vi "PIDBoundaries.vi"(0 "SetPointIn":dbl[](array[numeric]), 1 "EncPosIn":dbl[](array[numeric]), 2 "BndrsCluster":T2, 3 "PIDGainsIn":T1, 4 "EncMax":dbl[](array[numeric])) -> (5 "SetPointOut":dbl[](array[numeric]), 6 "PIDGainsOut":T3(array[cluster]))   [LabVIEW 2013]
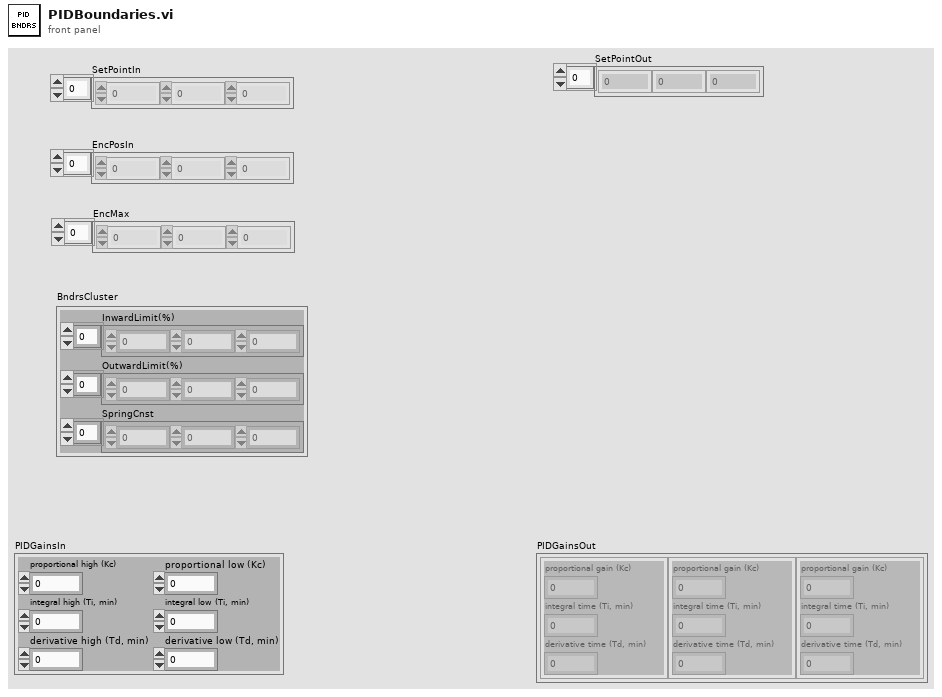
[diagram p1: front panel]
types:
  T1 = cluster{"proportional high (Kc)":dbl, "integral high (Ti, min)":dbl, "derivative high (Td, min)":dbl, "derivative low (Td, min)":dbl, "integral low (Ti, min)":dbl, "proportional low (Kc)":dbl}
  T2 = cluster{"InwardLimit(%)":dbl[], "OutwardLimit(%)":dbl[], "SpringCnst":dbl[]}
  T3 = cluster{"proportional gain (Kc)":dbl, "integral time (Ti, min)":dbl, "derivative time (Td, min)":dbl}[]
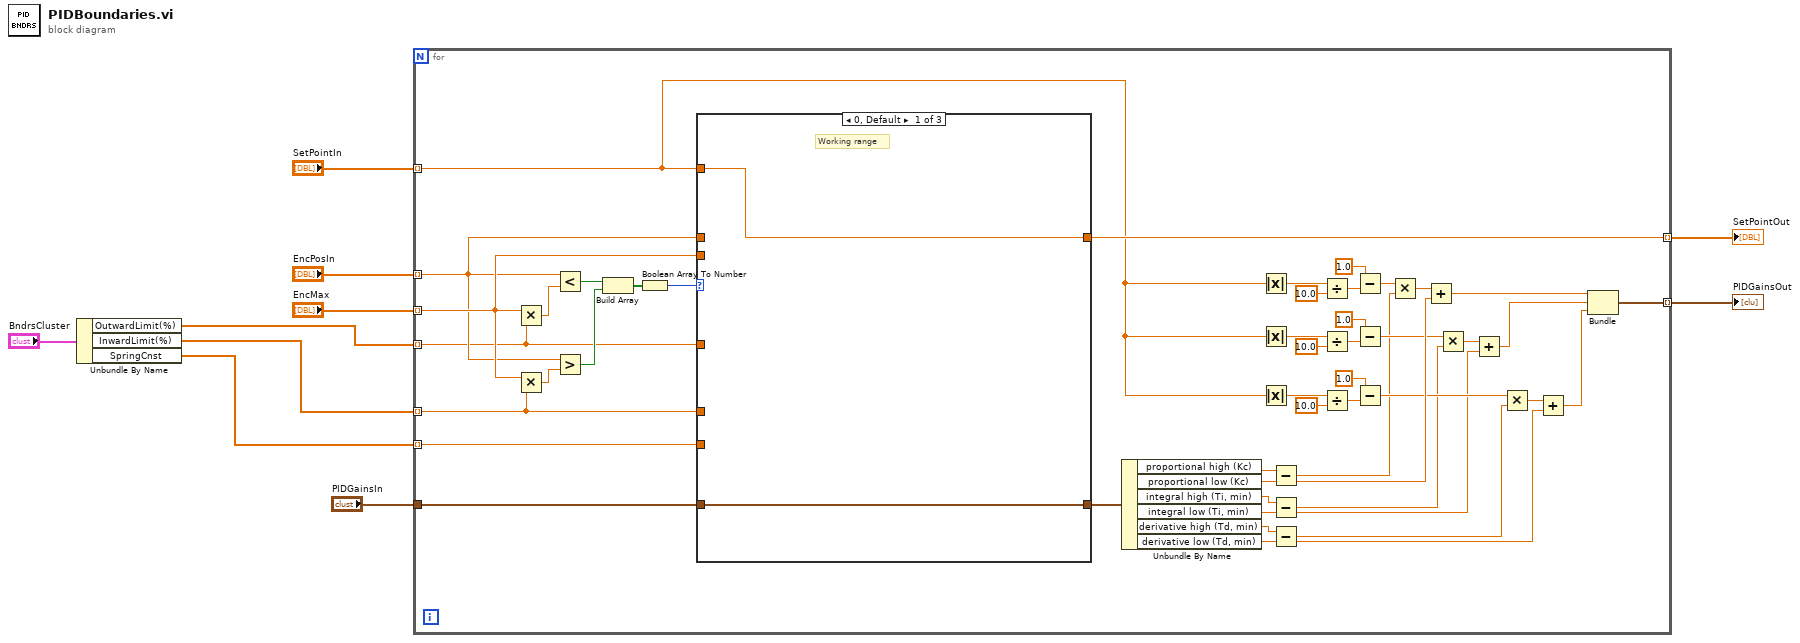
[diagram p0: block diagram]
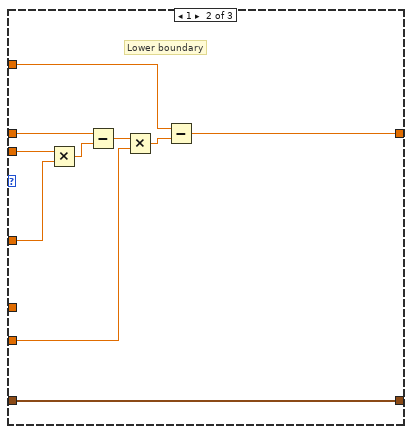
[diagram p2: hidden frame]
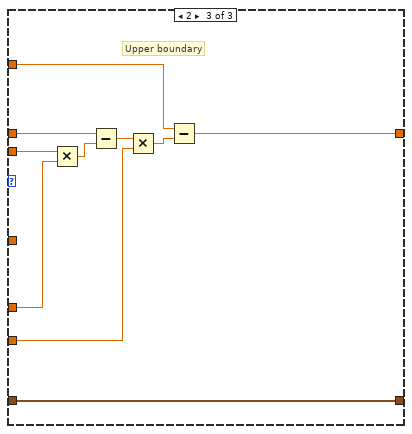
[diagram p3: hidden frame]
diagram:
  n1 = Unbundle By Name("BndrsCluster") -> ("OutwardLimit(%)"=w6:dbl[], "InwardLimit(%)"=w5:dbl[], "SpringCnst"=w4:dbl[])
  n2 = for {
    tunnel: "SetPointIn" -> [w22] mode=indexing
    tunnel: "EncMax" -> [w51] mode=indexing
    tunnel: "EncPosIn" -> [w50] mode=indexing
    tunnel: [w44] -> w10 mode=indexing
    tunnel: w6 -> [w49] mode=indexing
    tunnel: w5 -> [w48] mode=indexing
    tunnel: w4 -> [w47] mode=indexing
    tunnel: "PIDGainsIn" -> [w46]
    tunnel: [w11] -> w1 mode=indexing
    n3 = Multiply(x=w51, y=w49) -> (x*y=w56:dbl)
    n4 = Multiply(x=w51, y=w48) -> (x*y=w55:dbl)
    n5 = Less?(x=w50, y=w56) -> (x < y?=w54:bool)
    n6 = Greater?(x=w50, y=w55) -> (0:w53:bool)
    n7 = Build Array(w54, w53) -> (w52:bool[])
    n8 = Boolean Array To Number(Boolean array=w52) -> (number=w45:u32)
    n9 = case shown="0, Default" w45 {
      tunnel: [w57 w60 w70] -> w44
      tunnel: w22 -> [w57 w65 w77]
      tunnel: w50 -> [_ w64 w74]
      tunnel: w51 -> [_ w63 w73]
      tunnel: w46 -> [w58 w59 w69]
      tunnel: [w58 w59 w69] -> w38
      tunnel: w47 -> [_ w62 w72]
      tunnel: w49 -> [_ w61 _]
      tunnel: w48 -> [_ _ w71]
      frame 0, Default {
        # "Working range"
      }
      frame 1 {
        # "Lower boundary"
        n10 = Multiply(x=w63, y=w61) -> (x*y=w68:dbl)
        n11 = Subtract(x=w64, y=w68) -> (x-y=w67:dbl)
        n12 = Multiply(x=w67, y=w62) -> (x*y=w66:dbl)
        n13 = Subtract(x=w65, y=w66) -> (x-y=w60:dbl)
      }
      frame 2 {
        # "Upper boundary"
        n14 = Multiply(x=w73, y=w71) -> (x*y=w78:dbl)
        n15 = Subtract(x=w74, y=w78) -> (x-y=w76:dbl)
        n16 = Multiply(x=w76, y=w72) -> (x*y=w75:dbl)
        n17 = Subtract(x=w77, y=w75) -> (x-y=w70:dbl)
      }
    }
    n18 = Unbundle By Name(w38) -> ("proportional high (Kc)"=w37:dbl, "proportional low (Kc)"=w35:dbl, "integral high (Ti, min)"=w20:dbl, "integral low (Ti, min)"=w17:dbl, "derivative high (Td, min)"=w19:dbl, "derivative low (Td, min)"=w15:dbl)
    n19 = Absolute Value(x=w22) -> (abs(x)=w43:dbl)
    n20 = Absolute Value(x=w22) -> (abs(x)=w28:dbl)
    n21 = Absolute Value(x=w22) -> (abs(x)=w27:dbl)
    n22 = Subtract(x=w37, y=w35) -> (x-y=w21:dbl)
    n23 = Subtract(x=w20, y=w17) -> (x-y=w18:dbl)
    n24 = Subtract(x=w19, y=w15) -> (x-y=w16:dbl)
    n25 = Divide(x=w43, y=10.0) -> (x/y=w41:dbl)
    n26 = Divide(x=w28, y=10.0) -> (x/y=w30:dbl)
    n27 = Divide(x=w27, y=10.0) -> (x/y=w25:dbl)
    n28 = Subtract(x=1.0, y=w41) -> (x-y=w39:dbl)
    n29 = Subtract(x=1.0, y=w30) -> (x-y=w32:dbl)
    n30 = Subtract(x=1.0, y=w25) -> (x-y=w23:dbl)
    n31 = Multiply(x=w39, y=w21) -> (x*y=w36:dbl)
    n32 = Add(x=w36, y=w35) -> (x+y=w34:dbl)
    n33 = Multiply(x=w32, y=w18) -> (x*y=w33:dbl)
    n34 = Add(x=w33, y=w17) -> (x+y=w14:dbl)
    n35 = Multiply(x=w23, y=w16) -> (x*y=w13:dbl)
    n36 = Add(x=w13, y=w15) -> (x+y=w12:dbl)
    n37 = Bundle(w34, w14, w12) -> (w11:cluster{dbl, dbl, dbl})  [unwired: 1 in]
  }
  "SetPointOut" <- w10
  "PIDGainsOut" <- w1
